vi "PixelFormatEnumLookupTable.vi"(1 "pixel_format_enum":T1) -> (0 "pixel_format_integer":u32 format="%.0x")   [LabVIEW 2024, in "SDL3.lvlib" / "Render.lvlib"]
uses:
  Render.lvlib
  PixelFormat--enum.ctl
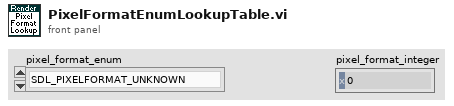
[diagram p1: front panel]
types:
  T1 = typedef "SDL3.lvlib/Render.lvlib/PixelFormat--enum.ctl" = enum32{"SDL_PIXELFORMAT_UNKNOWN", "SDL_PIXELFORMAT_INDEX1LSB", "SDL_PIXELFORMAT_INDEX1MSB", "SDL_PIXELFORMAT_INDEX2LSB", "SDL_PIXELFORMAT_INDEX2MSB", "SDL_PIXELFORMAT_INDEX4LSB", "SDL_PIXELFORMAT_INDEX4MSB", "SDL_PIXELFORMAT_INDEX8", "SDL_PIXELFORMAT_RGB332", "SDL_PIXELFORMAT_XRGB4444", "SDL_PIXELFORMAT_XBGR4444", "SDL_PIXELFORMAT_XRGB1555", "SDL_PIXELFORMAT_XBGR1555", "SDL_PIXELFORMAT_ARGB4444", "SDL_PIXELFORMAT_RGBA4444", "SDL_PIXELFORMAT_ABGR4444", "SDL_PIXELFORMAT_BGRA4444", "SDL_PIXELFORMAT_ARGB1555", "SDL_PIXELFORMAT_RGBA5551", "SDL_PIXELFORMAT_ABGR1555", "SDL_PIXELFORMAT_BGRA5551", "SDL_PIXELFORMAT_RGB565", "SDL_PIXELFORMAT_BGR565", "SDL_PIXELFORMAT_RGB24", "SDL_PIXELFORMAT_BGR24", "SDL_PIXELFORMAT_XRGB8888", "SDL_PIXELFORMAT_RGBX8888", "SDL_PIXELFORMAT_XBGR8888", "SDL_PIXELFORMAT_BGRX8888", "SDL_PIXELFORMAT_ARGB8888", "SDL_PIXELFORMAT_RGBA8888", "SDL_PIXELFORMAT_ABGR8888", "SDL_PIXELFORMAT_BGRA8888", "SDL_PIXELFORMAT_XRGB2101010", "SDL_PIXELFORMAT_XBGR2101010", "SDL_PIXELFORMAT_ARGB2101010", "SDL_PIXELFORMAT_ABGR2101010", "SDL_PIXELFORMAT_RGB48", "SDL_PIXELFORMAT_BGR48", "SDL_PIXELFORMAT_RGBA64", "SDL_PIXELFORMAT_ARGB64", "SDL_PIXELFORMAT_BGRA64", "SDL_PIXELFORMAT_ABGR64", "SDL_PIXELFORMAT_RGB48_FLOAT", "SDL_PIXELFORMAT_BGR48_FLOAT", "SDL_PIXELFORMAT_RGBA64_FLOAT", "SDL_PIXELFORMAT_ARGB64_FLOAT", "SDL_PIXELFORMAT_BGRA64_FLOAT", "SDL_PIXELFORMAT_ABGR64_FLOAT", "SDL_PIXELFORMAT_RGB96_FLOAT", "SDL_PIXELFORMAT_BGR96_FLOAT", "SDL_PIXELFORMAT_RGBA128_FLOAT", "SDL_PIXELFORMAT_ARGB128_FLOAT", "SDL_PIXELFORMAT_BGRA128_FLOAT", "SDL_PIXELFORMAT_ABGR128_FLOAT"}
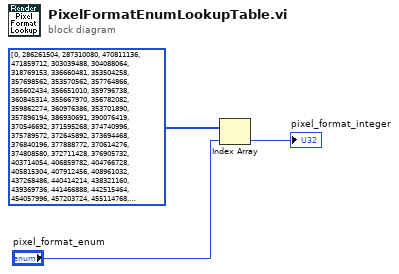
[diagram p0: block diagram]
diagram:
  n1 = Index Array(array=u32[] [0, 286261504, 287310080, 470811136, 471859712, 303039488, 304088064, 318769153, 336660481, 353504258, 357698562, 353570562, 357764866, 355602434, 356651010, 359796738, 360845314, 355667970, 356782082, 359862274, 360976386, 353701890, 357896194, 386930691, 390076419, 370546692, 371595268, 374740996, 375789572, 372645892, 373694468, 376840196, 377888772, 370614276, 374808580, 372711428, 376905732, 403714054, 406859782, 404766728, 405815304, 407912456, 408961032, 437268486, 440414214, 438321160, 439369736, 441466888, 442515464, 454057996, 457203724, 455114768, 456163344, 458260496, 459309072] ("Lookup"), index="pixel_format_enum") -> (element=→"pixel_format_integer":u32)
